vi "LB_FocusNameArray_Tests.vi"(11 "error in":errorcluster) -> (15 "error out":errorcluster)   [LabVIEW 2016, in "DronaTest.lvlib"]
uses:
  DronaTest.lvlib
  APIs/Stimulus/ControlValue/typedef/Name&Occurrence.ctl
  APIs/Stimulus/ControlValue/SetValueAuto.vi
  APIs/Stimulus/ControlValue/Controls/Listbox/SetValueByArrayName.vi
  APIs/Assert/AssertControlValue/Controls/Listbox/AssertValueByArrayName.vi
  <vilib>/addons/_JKI Toolkits/Caraya/classes/Assert/Assert Error.vi
  <vilib>/addons/_JKI Toolkits/Caraya/classes/Assert/Assert Equal Value_Variant.vi
  <vilib>/addons/_JKI Toolkits/Caraya/classes/Test/Test.lvclass
  Drona.lvlib
  <vilib>/SLL Toolkit/SLL Debug/SLL Debug.lvlib
  <vilib>/addons/_JKI Toolkits/Caraya/classes/Assert/Assert.lvclass
  APIs/Stimulus/ControlValue/Controls/Listbox/StimulusListbox.lvlib
  APIs/Assert/AssertControlValue/Controls/Listbox/AssertListbox.lvlib
  APIs/Stimulus/ControlValue/ControlValue.lvlib
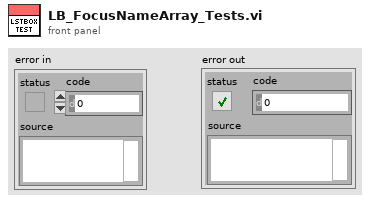
[diagram p1: front panel]
types:
  T1 = typedef "Drona.lvlib/ControlValue.lvlib/Name&Occurrence.ctl" = cluster{"ItemName":string, "Occurrence":i32}
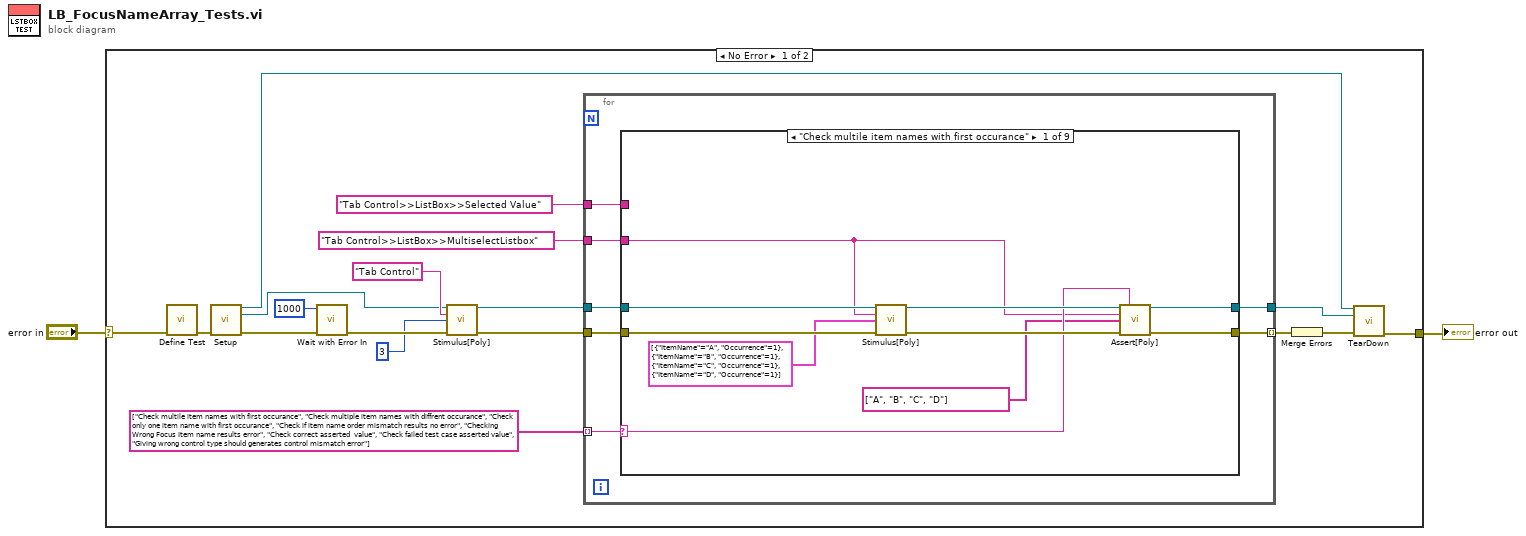
[diagram p0: block diagram]
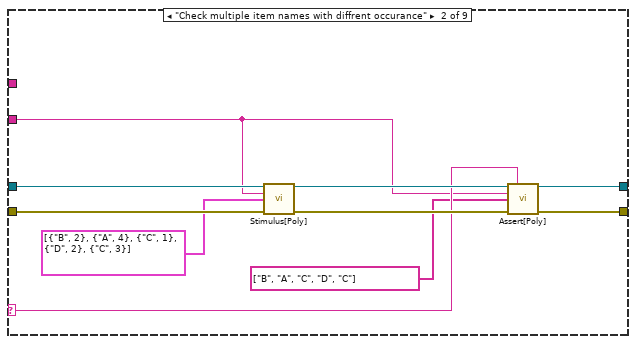
[diagram p2: hidden frame]
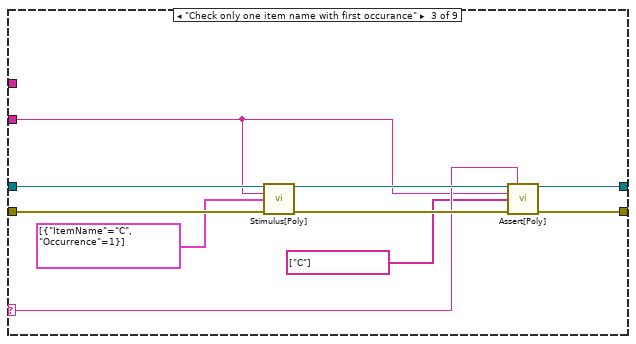
[diagram p3: hidden frame]
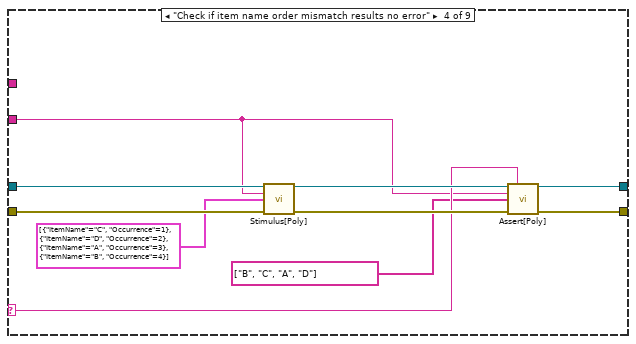
[diagram p4: hidden frame]
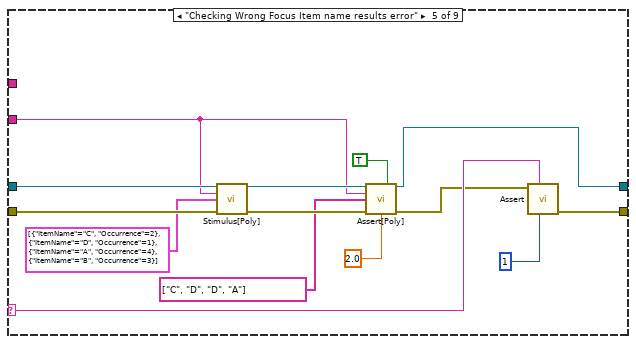
[diagram p5: hidden frame]
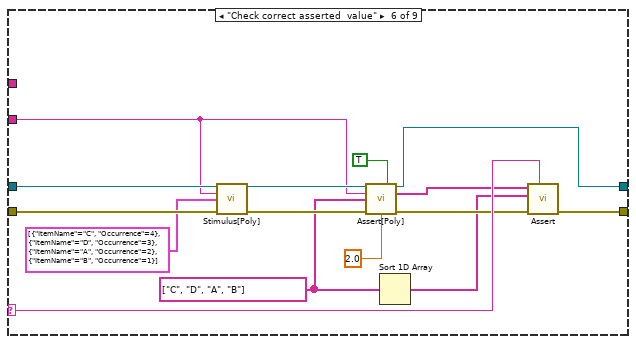
[diagram p6: hidden frame]
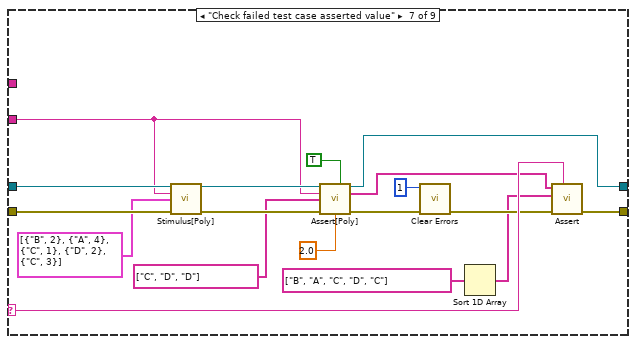
[diagram p7: hidden frame]
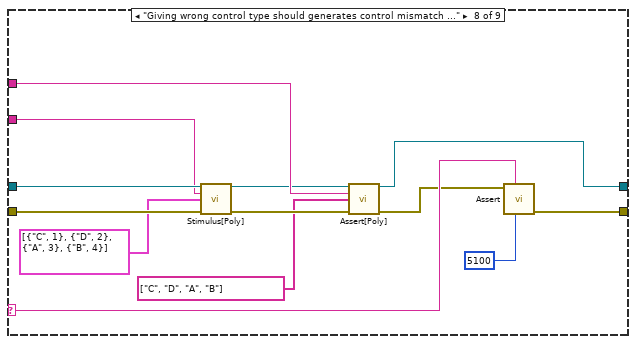
[diagram p8: hidden frame]
diagram:
  n1 = case shown="No Error" "error in" {
    selector: "error in" -> [w20 w130]
    tunnel: [w3 w130] -> w1
    frame No Error {
      n2 = call <vilib>:"Define Test.vi"("error in (no error)"=w20) -> ("error out"=w9:errorcluster)  [unwired: 9 in, 1 out]
      n3 = call "Setup.vi"("error in"=w9) -> ("Application Ref"=w5:refnum<vi>, "VI out"=w7:refnum<vi>, "error out"=w8:errorcluster)  [unwired: 12 in]
      n4 = call <vilib>:"Wait with Error In.vi"("error in (no error)"=w8, "milliseconds to wait"=u32 1000) -> ("error out"=w18:errorcluster)  [unwired: 9 in]
      n5 = call-poly "Stimulus[Poly].vi"("VI Reference In"=w7, "Control Path"="Tab Control", "Value (Signaling)"=3, "error in"=w18) -> ("VI Reference Out"=w14:refnum<vi>, "error out"=w17:errorcluster)  [unwired: 10 in]
      n6 = for {
        tunnel: w14 -> [w26]
        tunnel: "Tab Control>>ListBox>>MultiselectListbox" ("Control Path") -> [w25]
        tunnel: "Tab Control>>ListBox>>Selected Value" ("Control Path") -> [w24]
        tunnel: string[] ["Check multile item names with first occurance", "Check multiple item names with diffrent occurance", "Check only one item name with first occurance", "Check if item name order mismatch results no error", "Checking Wrong Focus Item name results error", "Check correct asserted  value", "Check failed test case asserted value", "Giving wrong control type should generates control mismatch error"] -> [w22] mode=indexing
        tunnel: [w21] -> w4
        tunnel: w17 -> [w27]
        tunnel: [w23] -> w10 mode=indexing
        n7 = case shown="\"Check multile item names with first occurance\"" w22 {
          selector: w22 -> [w31 w41 w51 w61 w80 w95 w113 w126 _]
          tunnel: w27 -> [w37 w47 w57 w67 w78 w94 w112 w121 w129]
          tunnel: w26 -> [w36 w46 w56 w66 w77 w93 w111 w119 w128]
          tunnel: w25 -> [w30 w40 w50 w60 w74 w90 w108 w117 _]
          tunnel: w24 -> [_ _ _ _ _ _ _ w123 _]
          tunnel: [w33 w43 w53 w63 w81 w96 w114 w127 w129] -> w23
          tunnel: [w32 w42 w52 w62 w73 w89 w107 w122 w128] -> w21
          frame "Check multile item names with first occurance" {
            n8 = call-poly "Stimulus[Poly].vi"("VI Reference In"=w36, "Control Path"=w30, "Name Array"=T1[] [{"ItemName"="A", "Occurrence"=1}, {"ItemName"="B", "Occurrence"=1}, {"ItemName"="C", "Occurrence"=1}, {"ItemName"="D", "Occurrence"=1}], "Error In"=w37) -> ("VI Reference Out"=w34:refnum<vi>, "Error Out"=w35:errorcluster)  [unwired: 10 in]
            n9 = call-poly "Assert[Poly].vi"("VI Reference In"=w34, "Test Label"=w31, "Control Path"=w30, "Focus Item Names"=string[] ["A", "B", "C", "D"], "Error In"=w35) -> ("VI Reference Out"=w32:refnum<vi>, "Error Out"=w33:errorcluster)  [unwired: 8 in, 1 out]
          }
          frame "Check multiple item names with diffrent occurance" {
            n10 = call-poly "Stimulus[Poly].vi"("VI Reference In"=w46, "Control Path"=w40, "Name Array"=T1[] [{"ItemName"="B", "Occurrence"=2}, {"ItemName"="A", "Occurrence"=4}, {"ItemName"="C", "Occurrence"=1}, {"ItemName"="D", "Occurrence"=2}, {"ItemName"="C", "Occurrence"=3}], "Error In"=w47) -> ("VI Reference Out"=w44:refnum<vi>, "Error Out"=w45:errorcluster)  [unwired: 10 in]
            n11 = call-poly "Assert[Poly].vi"("VI Reference In"=w44, "Test Label"=w41, "Control Path"=w40, "Focus Item Names"=string[] ["B", "A", "C", "D", "C"], "Error In"=w45) -> ("VI Reference Out"=w42:refnum<vi>, "Error Out"=w43:errorcluster)  [unwired: 8 in, 1 out]
          }
          frame "Check only one item name with first occurance" {
            n12 = call-poly "Stimulus[Poly].vi"("VI Reference In"=w56, "Control Path"=w50, "Name Array"=T1[] [{"ItemName"="C", "Occurrence"=1}], "Error In"=w57) -> ("VI Reference Out"=w54:refnum<vi>, "Error Out"=w55:errorcluster)  [unwired: 10 in]
            n13 = call-poly "Assert[Poly].vi"("VI Reference In"=w54, "Test Label"=w51, "Control Path"=w50, "Focus Item Names"=string[] ["C"], "Error In"=w55) -> ("VI Reference Out"=w52:refnum<vi>, "Error Out"=w53:errorcluster)  [unwired: 8 in, 1 out]
          }
          frame "Check if item name order mismatch results no error" {
            n14 = call-poly "Stimulus[Poly].vi"("VI Reference In"=w66, "Control Path"=w60, "Name Array"=T1[] [{"ItemName"="C", "Occurrence"=1}, {"ItemName"="D", "Occurrence"=2}, {"ItemName"="A", "Occurrence"=3}, {"ItemName"="B", "Occurrence"=4}], "Error In"=w67) -> ("VI Reference Out"=w64:refnum<vi>, "Error Out"=w65:errorcluster)  [unwired: 10 in]
            n15 = call-poly "Assert[Poly].vi"("VI Reference In"=w64, "Test Label"=w61, "Control Path"=w60, "Focus Item Names"=string[] ["B", "C", "A", "D"], "Error In"=w65) -> ("VI Reference Out"=w62:refnum<vi>, "Error Out"=w63:errorcluster)  [unwired: 8 in, 1 out]
          }
          frame "Checking Wrong Focus Item name results error" {
            n16 = call-poly "Stimulus[Poly].vi"("VI Reference In"=w77, "Control Path"=w74, "Name Array"=T1[] [{"ItemName"="C", "Occurrence"=2}, {"ItemName"="D", "Occurrence"=1}, {"ItemName"="A", "Occurrence"=4}, {"ItemName"="B", "Occurrence"=3}], "Error In"=w78) -> ("VI Reference Out"=w75:refnum<vi>, "Error Out"=w76:errorcluster)  [unwired: 10 in]
            n17 = call-poly "Assert[Poly].vi"("VI Reference In"=w75, "Assert Only? (F)"=TRUE, "Control Path"=w74, "Focus Item Names"=string[] ["C", "D", "D", "A"], "Error In"=w76, "Timeout(5 sec)"=2.0) -> ("VI Reference Out"=w73:refnum<vi>, "Error Out"=w72:errorcluster)  [unwired: 7 in, 1 out]
            n18 = call-poly <vilib>:"Assert.vi"("error code (1)"=1, "Label"=w80, "Error?"=w72) -> ("error out"=w81:errorcluster)  [unwired: 7 in, 1 out]
          }
          frame "Check correct asserted  value" {
            w83 = string[] ["C", "D", "A", "B"] ("Focus Item Names")
            n19 = call-poly "Stimulus[Poly].vi"("VI Reference In"=w93, "Control Path"=w90, "Name Array"=T1[] [{"ItemName"="C", "Occurrence"=4}, {"ItemName"="D", "Occurrence"=3}, {"ItemName"="A", "Occurrence"=2}, {"ItemName"="B", "Occurrence"=1}], "Error In"=w94) -> ("VI Reference Out"=w91:refnum<vi>, "Error Out"=w92:errorcluster)  [unwired: 10 in]
            n20 = call-poly "Assert[Poly].vi"("VI Reference In"=w91, "Assert Only? (F)"=TRUE, "Control Path"=w90, "Focus Item Names"=w83, "Error In"=w92, "Timeout(5 sec)"=2.0) -> ("VI Reference Out"=w89:refnum<vi>, "Asserted Value"=w84:string[], "Error Out"=w85:errorcluster)  [unwired: 7 in]
            n21 = Sort 1D Array(array=w83) -> (sorted array=w82:string[])
            n22 = call-poly <vilib>:"Assert.vi"("Label"=w95, "error in (no error)"=w85, "Y"=w82, "X"=w84) -> ("error out"=w96:errorcluster)  [unwired: 6 in, 1 out]
          }
          frame "Check failed test case asserted value" {
            n23 = call-poly "Stimulus[Poly].vi"("VI Reference In"=w111, "Control Path"=w108, "Name Array"=T1[] [{"ItemName"="B", "Occurrence"=2}, {"ItemName"="A", "Occurrence"=4}, {"ItemName"="C", "Occurrence"=1}, {"ItemName"="D", "Occurrence"=2}, {"ItemName"="C", "Occurrence"=3}], "Error In"=w112) -> ("VI Reference Out"=w109:refnum<vi>, "Error Out"=w110:errorcluster)  [unwired: 10 in]
            n24 = call-poly "Assert[Poly].vi"("VI Reference In"=w109, "Assert Only? (F)"=TRUE, "Control Path"=w108, "Focus Item Names"=string[] ["C", "D", "D"], "Error In"=w110, "Timeout(5 sec)"=2.0) -> ("VI Reference Out"=w107:refnum<vi>, "Asserted Value"=w101:string[], "Error Out"=w106:errorcluster)  [unwired: 7 in]
            n25 = call <vilib>:"Clear Errors.vi"("error in (no error)"=w106, "specific error code to clear (0: all)"=1) -> ("error out"=w103:errorcluster)  [unwired: 4 in, 1 out]
            n26 = Sort 1D Array(array=string[] ["B", "A", "C", "D", "C"] ("Focus Item Names")) -> (sorted array=w97:string[])
            n27 = call-poly <vilib>:"Assert.vi"("Label"=w113, "error in (no error)"=w103, "Y"=w97, "X"=w101) -> ("error out"=w114:errorcluster)  [unwired: 6 in, 1 out]
          }
          frame "Giving wrong control type should generates control mismatch error" {
            n28 = call-poly "Stimulus[Poly].vi"("VI Reference In"=w119, "Control Path"=w117, "Name Array"=T1[] [{"ItemName"="C", "Occurrence"=1}, {"ItemName"="D", "Occurrence"=2}, {"ItemName"="A", "Occurrence"=3}, {"ItemName"="B", "Occurrence"=4}], "Error In"=w121) -> ("VI Reference Out"=w118:refnum<vi>, "Error Out"=w120:errorcluster)  [unwired: 10 in]
            n29 = call-poly "Assert[Poly].vi"("VI Reference In"=w118, "Control Path"=w123, "Focus Item Names"=string[] ["C", "D", "A", "B"], "Error In"=w120) -> ("VI Reference Out"=w122:refnum<vi>, "Error Out"=w124:errorcluster)  [unwired: 9 in, 1 out]
            n30 = call-poly <vilib>:"Assert.vi"("error code (1)"=5100, "Label"=w126, "Error?"=w124) -> ("error out"=w127:errorcluster)  [unwired: 7 in, 1 out]
          }
          frame Default {
          }
        }
      }
      n31 = Merge Errors(w10) -> (w6:errorcluster)
      n32 = call "TearDown.vi"("Application Ref"=w5, "VI in"=w4, "error in (no error)"=w6) -> ("error out"=w3:errorcluster)  [unwired: 12 in]
    }
    frame Error {
    }
  }
  "error out" <- w1
